vi "_builtins_icon_color.vi"(10 "Default Color (none)":u32=16777215 format="%08x", 11 "color (name, #ddeeff, ?)":string) -> (1 "Invert Text?":bool, 2 "Color":u32(colorbox), 3 "Found?":bool)   [LabVIEW 2019, in "Script.lvlib"]
doc: "Get color by X11 name (\"cyan\"), html hash code (\"#FFFFFF\") or random (\"?\"). Not all X11 colors are included because of LabVIEW's 24bit to 8bit icon compression."
uses:
  Script.lvlib
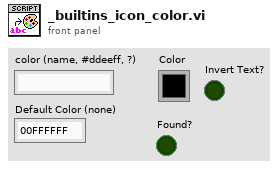
[diagram p1: front panel]
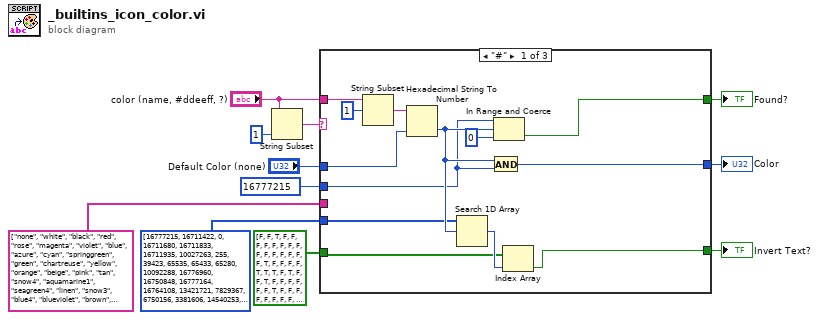
[diagram p0: block diagram]
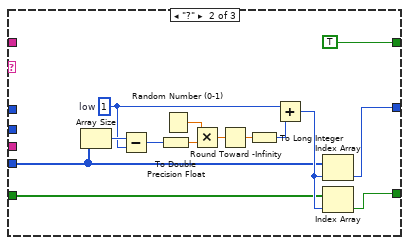
[diagram p2: hidden frame]
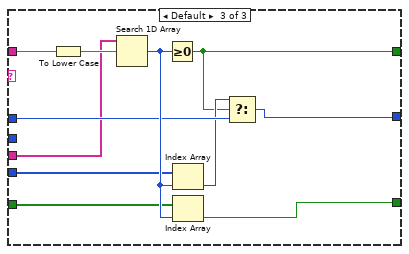
[diagram p3: hidden frame]
diagram:
  n1 = String Subset(string="color (name, #ddeeff, ?)", length (rest)=1 ("length (rest)")) -> (substring=w10:string)  [unwired: 1 in]
  n2 = case shown="\"#\"" w10 {
    tunnel: "color (name, #ddeeff, ?)" -> [w24 _ w49]
    tunnel: [w19 w35 w46] -> w8
    tunnel: [w20 w34 w48] -> w7
    tunnel: "Default Color (none)" -> [w13 _ w44]
    tunnel: [w16 TRUE w42] -> w5
    tunnel: bool[] [FALSE, FALSE, TRUE, FALSE, FALSE, FALSE, FALSE, FALSE, FALSE, FALSE, FALSE, FALSE, FALSE, FALSE, FALSE, FALSE, FALSE, FALSE, TRUE, FALSE, FALSE, FALSE, FALSE, TRUE, TRUE, TRUE, FALSE, TRUE, FALSE, FALSE, TRUE, FALSE, FALSE, FALSE, FALSE, FALSE, FALSE, TRUE, FALSE, FALSE, FALSE, FALSE, FALSE, FALSE, FALSE, FALSE, TRUE, TRUE, FALSE, TRUE, FALSE, FALSE, TRUE, FALSE, FALSE, TRUE, FALSE, FALSE, TRUE, FALSE, FALSE, FALSE, FALSE, TRUE, TRUE, TRUE, TRUE, TRUE, FALSE, FALSE, TRUE, TRUE, FALSE, TRUE, TRUE, FALSE, FALSE, FALSE, TRUE, TRUE, FALSE, FALSE, TRUE, FALSE, FALSE, FALSE, FALSE, TRUE, FALSE, FALSE, TRUE, FALSE, FALSE, FALSE, TRUE, FALSE, FALSE, TRUE, FALSE, TRUE, FALSE, FALSE, FALSE, FALSE, TRUE, FALSE, FALSE, FALSE, FALSE, TRUE, FALSE, FALSE, FALSE, FALSE, FALSE, FALSE, FALSE, TRUE, TRUE, FALSE, FALSE, TRUE, FALSE, FALSE, TRUE, FALSE, FALSE, FALSE, FALSE, TRUE, TRUE, TRUE, TRUE, FALSE, FALSE, FALSE, FALSE, FALSE, FALSE, FALSE, TRUE, FALSE, FALSE, FALSE, TRUE, FALSE, FALSE, FALSE, TRUE, FALSE] ("invert") -> [w14 w26 w39]
    tunnel: u32[] [16777215, 16711422, 0, 16711680, 16711833, 16711935, 10027263, 255, 39423, 65535, 65433, 65280, 10092288, 16776960, 16750848, 16777164, 16764108, 13421721, 7829367, 6750156, 3381606, 14540253, 13421772, 153, 10040268, 10040115, 16724787, 13382451, 16764057, 13408614, 10053222, 6723993, 10092543, 10079487, 6737100, 6749952, 6736896, 3381504, 13395507, 16737843, 16737894, 6724095, 52428, 39321, 13408512, 16763904, 10053120, 26112, 13421670, 6710835, 13434726, 10079334, 6723891, 16737792, 13395456, 10040064, 13382655, 10040319, 6697881, 16750950, 10079385, 13434828, 6723942, 3355545, 4473924, 10027212, 13369446, 10027110, 52479, 39372, 26265, 6710886, 3381759, 26316, 3381555, 13408563, 16763955, 11184810, 1118481, 3355443, 10066329, 52224, 39168, 10092339, 16737996, 16737945, 13395609, 10040166, 13395558, 16777113, 10066278, 13434879, 10079436, 16751001, 10066227, 16751052, 13408665, 10053171, 3381657, 6710937, 10053375, 13421823, 3394611, 13369548, 10027161, 16724940, 16724889, 13382553, 6737049, 204, 13395660, 13395711, 10053324, 10066431, 3394662, 6711039, 3394764, 13369497, 102, 13434675, 16724736, 13382400, 16751103, 16738047, 10040217, 10092441, 6736998, 13408716, 16764159, 10053273, 6697932, 13369344, 10027008, 3368652, 3368703, 6750105, 3394713, 16750899, 6737151, 6724044, 3368601, 6710988, 65382, 52326, 39219, 3381708, 13382502, 13421568, 10066176, 10079283] ("bg") -> [w15 w25 w40]
    tunnel: string[] ["none", "white", "black", "red", "rose", "magenta", "violet", "blue", "azure", "cyan", "springgreen", "green", "chartreuse", "yellow", "orange", "beige", "pink", "tan", "snow4", "aquamarine1", "seagreen4", "linen", "snow3", "blue4", "blueviolet", "brown", "brown1", "brown3", "light", "burlywood3", "pink4", "cadetblue", "cadetblue1", "skyblue", "cadetblue3", "lawngreen", "chartreuse3", "chartreuse4", "coral3", "sienna2", "coral", "steelblue2", "cyan3", "cyan4", "gold3", "gold1", "gold4", "darkgreen", "khaki3", "darkolivegreen", "darkolivegreen1", "darkolivegreen3", "olivedrab", "darkorange1", "darkorange3", "orangered4", "darkorchid1", "purple", "purple4", "tan1", "darkseagreen", "darkseagreen1", "palegreen4", "royalblue4", "gray25", "darkviolet", "deeppink3", "deeppink4", "turquoise2", "deepskyblue3", "dodgerblue4", "gray35", "dodgerblue1", "dodgerblue3", "forestgreen", "tan3", "goldenrod1", "gray", "gray5", "gray15", "gray55", "green3", "green4", "greenyellow", "hotpink", "hotpink2", "pale", "maroon", "salmon3", "khaki", "khaki4", "lightblue1", "lightblue3", "lightcoral", "lightgoldenrod4", "pink2", "pink3", "tan4", "lightseagreen", "lightskyblue4", "slateblue1", "slategray1", "limegreen", "magenta3", "magenta4", "maroon1", "maroon2", "maroon3", "medium", "mediumblue", "orchid", "mediumorchid1", "mediumpurple", "mediumpurple1", "mediumseagreen", "slateblue2", "turquoise", "mediumvioletred", "midnightblue", "olivedrab1", "orangered1", "orangered3", "plum2", "orchid2", "orchid4", "palegreen", "palegreen3", "plum", "plum1", "plum4", "purple3", "red3", "red4", "royalblue", "royalblue1", "seagreen1", "seagreen3", "tan2", "skyblue2", "skyblue3", "skyblue4", "slateblue", "springgreen1", "springgreen3", "springgreen4", "steelblue", "violetred3", "yellow3", "yellow4", "yellowgreen"] ("name") -> [_ _ w41]
    tunnel: u32 16777215 -> [w12 _ _]
    frame "#" {
      n3 = String Subset(string=w24, offset (0)=1) -> (substring=w22:string)  [unwired: 1 in]
      n4 = Hexadecimal String To Number(string=w22, default (0uL)=w13) -> (number=w18:u32)  [unwired: 1 in, 1 out]
      n5 = Search 1D Array(1D array=w15, element=w18) -> (index of element=w21:i32)  [unwired: 1 in]
      n6 = And(x=w18, y=w12) -> (x .and. y?=w19:u32)
      n7 = In Range and Coerce(upper limit=w12, x=w18, lower limit=u32 0) -> (In Range?=w16:bool)  [unwired: 1 out]
      n8 = Index Array(array=w14, index=w21) -> (element=w20:bool)
    }
    frame "?" {
      w28 = 1  # low
      n9 = Array Size(array=w25) -> (size(s)=w32:i32)
      n10 = Subtract(x=w32, y=w28) -> (x-y=w31:i32)
      n11 = To Double Precision Float(number=w31) -> (double precision float=w38:dbl)
      n12 = Random Number (0-1)() -> (number: 0 to 1=w37:dbl)
      n13 = Multiply(x=w37, y=w38) -> (x*y=w36:dbl)
      n14 = Round Toward -Infinity(1:w36) -> (0:w30:dbl)
      n15 = To Long Integer(number=w30) -> (32bit integer=w29:i32)
      n16 = Add(x=w28, y=w29) -> (x+y=w27:i32)
      n17 = Index Array(array=w25, index=w27) -> (element=w35:u32)
      n18 = Index Array(array=w26, index=w27) -> (element=w34:bool)
    }
    frame Default {
      n19 = To Lower Case(string=w49) -> (all lower case string=w45:string)
      n20 = Search 1D Array(1D array=w41, element=w45) -> (index of element=w47:i32)  [unwired: 1 in]
      n21 = Greater Or Equal To 0?(x=w47) -> (x >= 0?=w42:bool)
      n22 = Index Array(array=w40, index=w47) -> (element=w43:u32)
      n23 = Index Array(array=w39, index=w47) -> (element=w48:bool)
      n24 = Select(t=w43, s=w42, f=w44) -> (s? t:f=w46:u32)
    }
  }
  "Color" <- w8
  "Invert Text?" <- w7
  "Found?" <- w5
